vi "TSCANFD_Write.vi"(8 "错误输入（无错误）":errorcluster, 10 "TCANFD":T1 {"AIsData" items=["数据帧", "远程帧"]; "AIsStd" items=["标准帧", "扩展帧"]; "AId" format="%x"; "AIdxchn" items=["CHN1", "CHN2", "CHN3", "CHN4", "CHN5", "CHN6", "CHN7", "CHN8", "CHN9", "CHN10", "CHN11", "CHN12", "CHN13", "CHN14", "CHN15", "CHN16", "CHN17", "CHN18", "CHN19", "CHN20", "CHN21", "CHN22", "CHN23", "CHN24", "CHN25", "CHN26", "CHN27", "CHN28", "CHN29", "CHN30", "CHN31", "CHN32"]}, 11 "路径输入":path) -> (0 "错误输出":errorcluster, 3 "路径输出":path)   [LabVIEW 2019]
uses:
  Typedef/TLibCANFD.ctl
panel:
  out "tsapp_transmit_can_async":i32
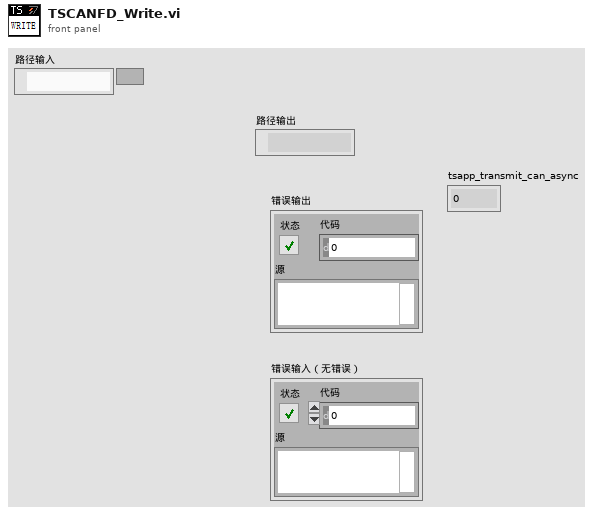
[diagram p1: front panel]
types:
  T1 = typedef "TLibCANFD.ctl" = cluster{"AIdxchn":u8, "AId":i32, "AIsStd":u8, "AIsData":u8, "ADLC":u8, "AIsFD":enum16{"Classic CAN报文", "FD CAN报文"}, "FDatas":cluster{"初始化的数组[0]":u8, "初始化的数组[1]":u8, "初始化的数组[2]":u8, "初始化的数组[3]":u8, "初始化的数组[4]":u8, "初始化的数组[5]":u8, "初始化的数组[6]":u8, "初始化的数组[7]":u8, "初始化的数组[8]":u8, "初始化的数组[9]":u8, "初始化的数组[10]":u8, "初始化的数组[11]":u8, "初始化的数组[12]":u8, "初始化的数组[13]":u8, "初始化的数组[14]":u8, "初始化的数组[15]":u8, "初始化的数组[16]":u8, "初始化的数组[17]":u8, "初始化的数组[18]":u8, "初始化的数组[19]":u8, "初始化的数组[20]":u8, "初始化的数组[21]":u8, "初始化的数组[22]":u8, "初始化的数组[23]":u8, "初始化的数组[24]":u8, "初始化的数组[25]":u8, "初始化的数组[26]":u8, "初始化的数组[27]":u8, "初始化的数组[28]":u8, "初始化的数组[29]":u8, "初始化的数组[30]":u8, "初始化的数组[31]":u8, "初始化的数组[32]":u8, "初始化的数组[33]":u8, "初始化的数组[34]":u8, "初始化的数组[35]":u8, "初始化的数组[36]":u8, "初始化的数组[37]":u8, "初始化的数组[38]":u8, "初始化的数组[39]":u8, "初始化的数组[40]":u8, "初始化的数组[41]":u8, "初始化的数组[42]":u8, "初始化的数组[43]":u8, "初始化的数组[44]":u8, "初始化的数组[45]":u8, "初始化的数组[46]":u8, "初始化的数组[47]":u8, "初始化的数组[48]":u8, "初始化的数组[49]":u8, "初始化的数组[50]":u8, "初始化的数组[51]":u8, "初始化的数组[52]":u8, "初始化的数组[53]":u8, "初始化的数组[54]":u8, "初始化的数组[55]":u8, "初始化的数组[56]":u8, "初始化的数组[57]":u8, "初始化的数组[58]":u8, "初始化的数组[59]":u8, "初始化的数组[60]":u8, "初始化的数组[61]":u8, "初始化的数组[62]":u8, "初始化的数组[63]":u8, "初始化的数组[64] ":u8}}
  T2 = cluster{"FIdxChn":u8, "FProperties":u8, "FDLC":u8, "FReserved":u8, "FIdentifier":i32, "FTimeUS":u64, "Fdata":cluster{"初始化的数组[0]":u8, "初始化的数组[1]":u8, "初始化的数组[2]":u8, "初始化的数组[3]":u8, "初始化的数组[4]":u8, "初始化的数组[5]":u8, "初始化的数组[6]":u8, "初始化的数组[7]":u8, "初始化的数组[8]":u8, "初始化的数组[9]":u8, "初始化的数组[10]":u8, "初始化的数组[11]":u8, "初始化的数组[12]":u8, "初始化的数组[13]":u8, "初始化的数组[14]":u8, "初始化的数组[15]":u8, "初始化的数组[16]":u8, "初始化的数组[17]":u8, "初始化的数组[18]":u8, "初始化的数组[19]":u8, "初始化的数组[20]":u8, "初始化的数组[21]":u8, "初始化的数组[22]":u8, "初始化的数组[23]":u8, "初始化的数组[24]":u8, "初始化的数组[25]":u8, "初始化的数组[26]":u8, "初始化的数组[27]":u8, "初始化的数组[28]":u8, "初始化的数组[29]":u8, "初始化的数组[30]":u8, "初始化的数组[31]":u8, "初始化的数组[32]":u8, "初始化的数组[33]":u8, "初始化的数组[34]":u8, "初始化的数组[35]":u8, "初始化的数组[36]":u8, "初始化的数组[37]":u8, "初始化的数组[38]":u8, "初始化的数组[39]":u8, "初始化的数组[40]":u8, "初始化的数组[41]":u8, "初始化的数组[42]":u8, "初始化的数组[43]":u8, "初始化的数组[44]":u8, "初始化的数组[45]":u8, "初始化的数组[46]":u8, "初始化的数组[47]":u8, "初始化的数组[48]":u8, "初始化的数组[49]":u8, "初始化的数组[50]":u8, "初始化的数组[51]":u8, "初始化的数组[52]":u8, "初始化的数组[53]":u8, "初始化的数组[54]":u8, "初始化的数组[55]":u8, "初始化的数组[56]":u8, "初始化的数组[57]":u8, "初始化的数组[58]":u8, "初始化的数组[59]":u8, "初始化的数组[60]":u8, "初始化的数组[61]":u8, "初始化的数组[62]":u8, "初始化的数组[63]":u8, "初始化的数组[64]":u8}}
  T3 = cluster{"初始化的数组[0]":u8, "初始化的数组[1]":u8, "初始化的数组[2]":u8, "初始化的数组[3]":u8, "初始化的数组[4]":u8, "初始化的数组[5]":u8, "初始化的数组[6]":u8, "初始化的数组[7]":u8, "初始化的数组[8]":u8, "初始化的数组[9]":u8, "初始化的数组[10]":u8, "初始化的数组[11]":u8, "初始化的数组[12]":u8, "初始化的数组[13]":u8, "初始化的数组[14]":u8, "初始化的数组[15]":u8, "初始化的数组[16]":u8, "初始化的数组[17]":u8, "初始化的数组[18]":u8, "初始化的数组[19]":u8, "初始化的数组[20]":u8, "初始化的数组[21]":u8, "初始化的数组[22]":u8, "初始化的数组[23]":u8, "初始化的数组[24]":u8, "初始化的数组[25]":u8, "初始化的数组[26]":u8, "初始化的数组[27]":u8, "初始化的数组[28]":u8, "初始化的数组[29]":u8, "初始化的数组[30]":u8, "初始化的数组[31]":u8, "初始化的数组[32]":u8, "初始化的数组[33]":u8, "初始化的数组[34]":u8, "初始化的数组[35]":u8, "初始化的数组[36]":u8, "初始化的数组[37]":u8, "初始化的数组[38]":u8, "初始化的数组[39]":u8, "初始化的数组[40]":u8, "初始化的数组[41]":u8, "初始化的数组[42]":u8, "初始化的数组[43]":u8, "初始化的数组[44]":u8, "初始化的数组[45]":u8, "初始化的数组[46]":u8, "初始化的数组[47]":u8, "初始化的数组[48]":u8, "初始化的数组[49]":u8, "初始化的数组[50]":u8, "初始化的数组[51]":u8, "初始化的数组[52]":u8, "初始化的数组[53]":u8, "初始化的数组[54]":u8, "初始化的数组[55]":u8, "初始化的数组[56]":u8, "初始化的数组[57]":u8, "初始化的数组[58]":u8, "初始化的数组[59]":u8, "初始化的数组[60]":u8, "初始化的数组[61]":u8, "初始化的数组[62]":u8, "初始化的数组[63]":u8, "初始化的数组[64] ":u8}
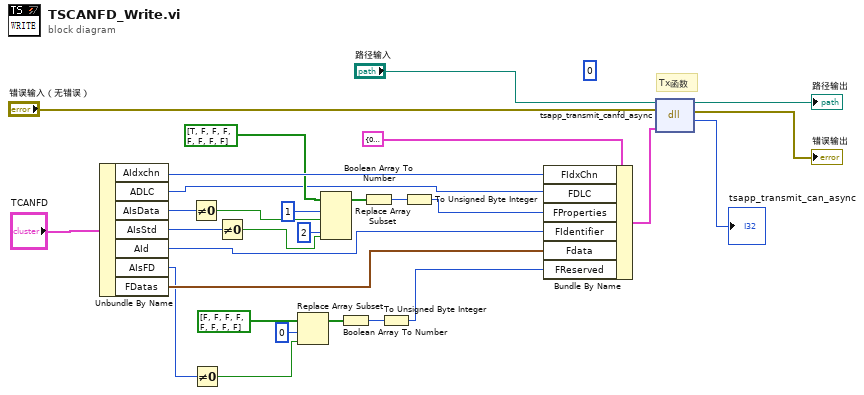
[diagram p0: block diagram]
diagram:
  (unwired) u8 0 ("FReserved")
  # "Tx函数"
  n1 = Unbundle By Name("TCANFD") -> ("AIdxchn"=w22:u8, "ADLC"=w12:u8, "AIsData"=w21:u8, "AIsStd"=w20:u8, "AId"=w23:i32, "AIsFD"=w3:enum16{"Classic CAN报文", "FD CAN报文"}, "FDatas"=w6:T3)
  n2 = Not Equal To 0?(x=w21) -> (x != 0?=w17:bool)
  n3 = Not Equal To 0?(x=w3) -> (x != 0?=w2:bool)
  n4 = Not Equal To 0?(x=w20) -> (x != 0?=w15:bool)
  n5 = Replace Array Subset(array=bool[] [FALSE, FALSE, FALSE, FALSE, FALSE, FALSE, FALSE, FALSE], new element=w2, index=0 ("索引")) -> (w4:bool[])
  n6 = Replace Array Subset(array=bool[] [TRUE, FALSE, FALSE, FALSE, FALSE, FALSE, FALSE, FALSE], new element #1=w17, index #1=1 ("索引"), new element #2=w15, index #2=2 ("索引")) -> (w14:bool[])
  n7 = Boolean Array To Number(Boolean array=w4) -> (number=w9:u32)
  n8 = Boolean Array To Number(Boolean array=w14) -> (number=w13:u32)
  n9 = To Unsigned Byte Integer(number=w9) -> (unsigned 8bit integer=w8:u8)
  n10 = To Unsigned Byte Integer(number=w13) -> (unsigned 8bit integer=w11:u8)
  n11 = Bundle By Name(cluster=T2 {"FIdxChn"=0, "FProperties"=0, "FDLC"=0, "FReserved"=0, "FIdentifier"=0, "FTimeUS"=0, "Fdata"={"初始化的数组[0]"=0, "初始化的数组[1]"=0, "初始化的数组[2]"=0, "初始化的数组[3]"=0, "初始化的数组[4]"=0, "初始化的数组[5]"=0, "初始化的数组[6]"=0, "初始化的数组[7]"=0, "初始化的数组[8]"=0, "初始化的数组[9]"=0, "初始化的数组[10]"=0, "初始化的数组[11]"=0, "初始化的数组[12]"=0, "初始化的数组[13]"=0, "初始化的数组[14]"=0, "初始化的数组[15]"=0, "初始化的数组[16]"=0, "初始化的数组[17]"=0, "初始化的数组[18]"=0, "初始化的数组[19]"=0, "初始化的数组[20]"=0, "初始化的数组[21]"=0, "初始化的数组[22]"=0, "初始化的数组[23]"=0, "初始化的数组[24]"=0, "初始化的数组[25]"=0, "初始化的数组[26]"=0, "初始化的数组[27]"=0, "初始化的数组[28]"=0, "初始化的数组[29]"=0, "初始化的数组[30]"=0, "初始化的数组[31]"=0, "初始化的数组[32]"=0, "初始化的数组[33]"=0, "初始化的数组[34]"=0, "初始化的数组[35]"=0, "初始化的数组[36]"=0, "初始化的数组[37]"=0, "初始化的数组[38]"=0, "初始化的数组[39]"=0, "初始化的数组[40]"=0, "初始化的数组[41]"=0, "初始化的数组[42]"=0, "初始化的数组[43]"=0, "初始化的数组[44]"=0, "初始化的数组[45]"=0, "初始化的数组[46]"=0, "初始化的数组[47]"=0, "初始化的数组[48]"=0, "初始化的数组[49]"=0, "初始化的数组[50]"=0, "初始化的数组[51]"=0, "初始化的数组[52]"=0, "初始化的数组[53]"=0, "初始化的数组[54]"=0, "初始化的数组[55]"=0, "初始化的数组[56]"=0, "初始化的数组[57]"=0, "初始化的数组[58]"=0, "初始化的数组[59]"=0, "初始化的数组[60]"=0, "初始化的数组[61]"=0, "初始化的数组[62]"=0, "初始化的数组[63]"=0, "初始化的数组[64]"=0}} ("ACAN"), "FIdxChn"=w22, "FDLC"=w12, "FProperties"=w11, "FIdentifier"=w23, "Fdata"=w6, "FReserved"=w8) -> (w25:T2)
  n12 = dll-call lib="PTH2@abs EDemo同星TSCAN_V1.2_20220228ConfigTSMaster.dll" fn="tsapp_transmit_canfd_async"(path in="路径输入", error in="错误输入（无错误）", "ACAN"=w25) -> (path out=→"路径输出":path, error out=→"错误输出":errorcluster, "tsapp_transmit_can_async"=→"tsapp_transmit_can_async":i32)  [unwired: 2 in]
